vi "Window-Export time series snippet.vi"(10 "New folder path":path, 11 "Existing AVI path":path) -> ()   [LabVIEW 2017]
uses:
  <vilib>/Utility/miscctls.llb/LVPointTypeDef.ctl
panel:
  out "Ended":bool
  out "Manually closed":bool
  out "Exporting snippet...":u8(slide) scale=0.0..100.0
  out "# of Frames in exported portion":i32 format="Number of frames: %.0f"
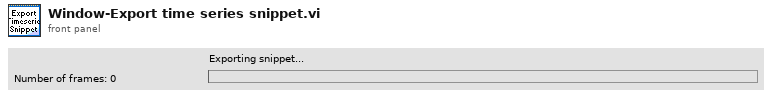
[diagram p1: front panel]
types:
  T1 = typedef "Image Type" = u32
  T2 = typedef "LVPointTypeDef.ctl" = cluster{"Horizontal":i16, "Vertical":i16}
  T3 = typedef "AVI modes refs cluster.ctl" = cluster{"AVI1 ref":T4, "AVI2 refs":T5[], "AVI # frames":u32[]}
  T4 = typedef "AviRefnum.ctl" = refnum<k1>
  T5 = typedef "IMAQ AVI2 Refnum.ctl" = refnum<k20>
  T6 = typedef "Fixed strings.ctl" = cluster{"ROI file name":string, "Normalised ROI file name":string, "Zplane Pockels values file name":string, "Functional data folder name":string, "Experiment Header file name":string, "Z-stack images folder name":string, "Groups setup rel. path":string, "Groups text file rel. path":string, "TDMS files folder name (F.img)":string, "TDMS files folder name (V.acq)":string, "TDMS files folder name (Pl.acq)":string, "Cycle rel times sequence file":string, "Dynamically called VIs folder name":string, "Time Series folder base name":string}
  T7 = typedef "IMAQ Image.ctl" = refnum<image>
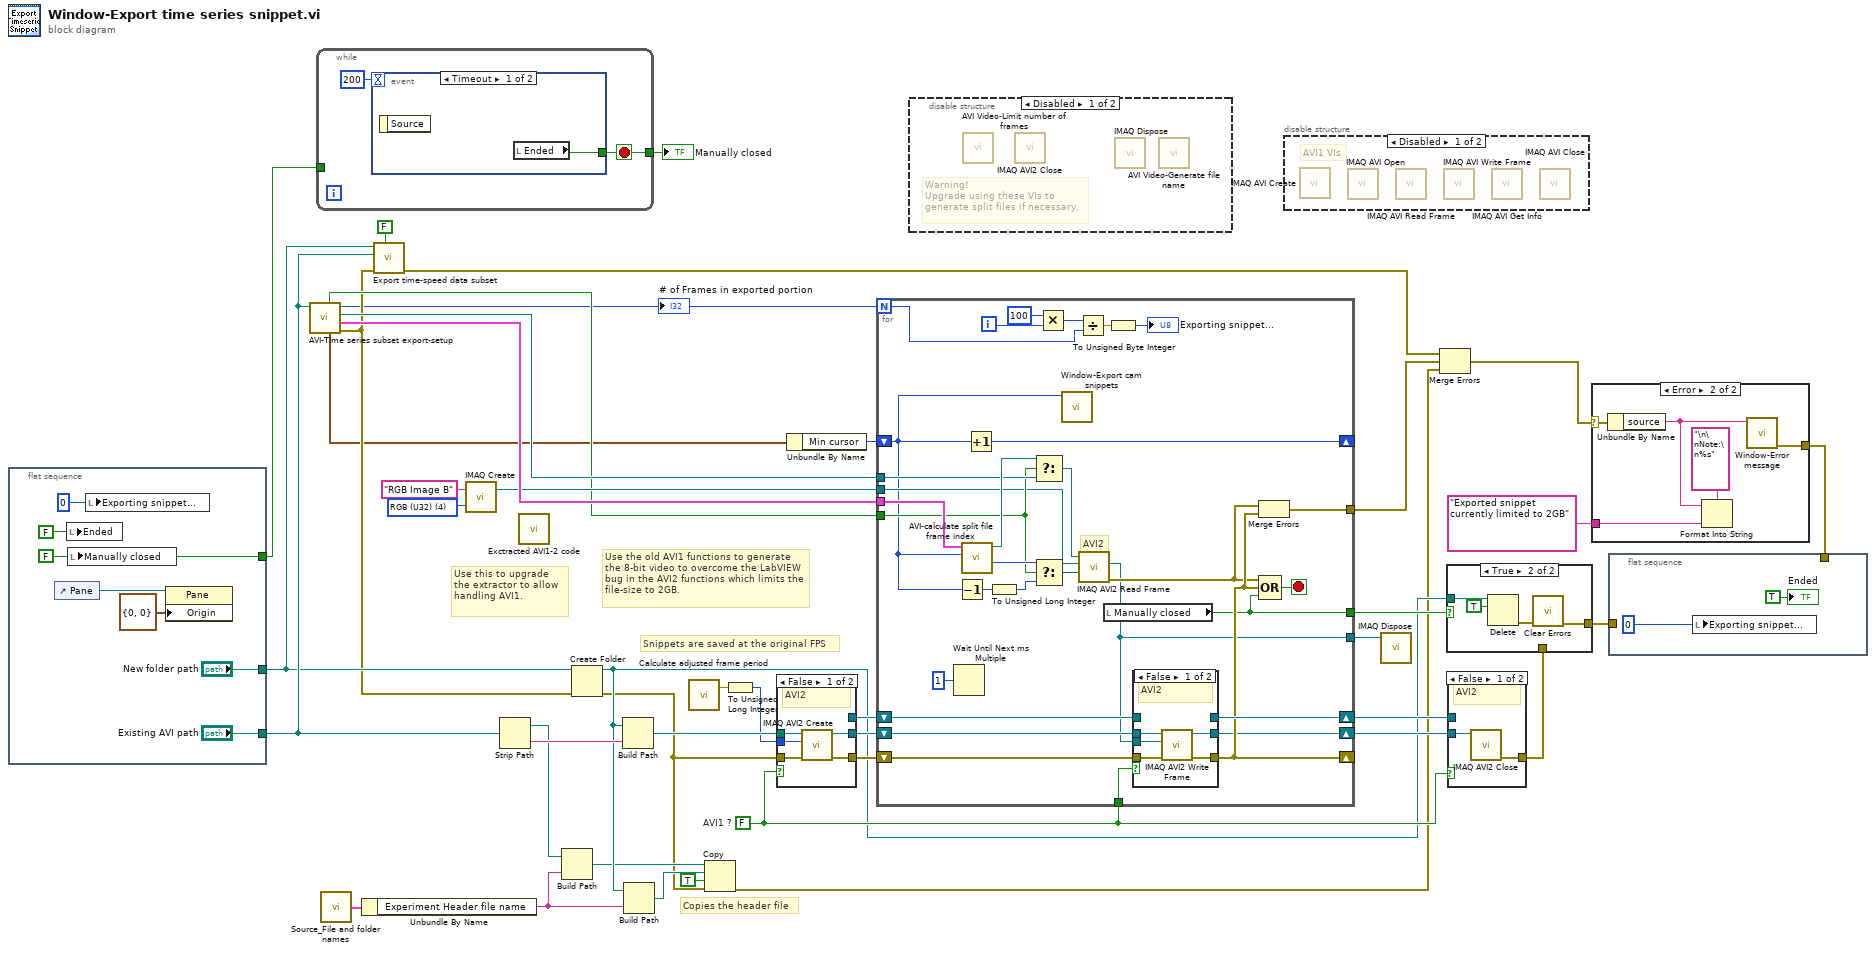
[diagram p0: block diagram]
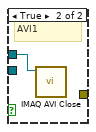
[diagram p4: hidden frame]
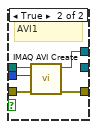
[diagram p5: hidden frame]
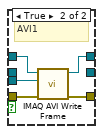
[diagram p6: hidden frame]
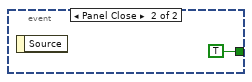
[diagram p8: hidden frame]
diagram:
  w30 = FALSE  # AVI1 ?
  w41 = T1 4 items=["Grayscale (U8)", "Grayscale (I16)", "Grayscale (SGL)", "Complex (CSG)", "RGB (U32)", "HSL (U32)", "RGB (U64)", "Grayscale (U16)"] ("Image Type")
  # "Snippets are saved at the original FPS"
  # "Use this to upgrade the extractor to allow handling AVI1."
  # "Copies the header file"
  # "Use the old AVI1 functions to generate the 8-bit video to overcome the LabVIEW bug in the AVI2 functions which limits the file-size to 2GB."
  n1 = flat-sequence {
    tunnel: ["Existing AVI path"] -> w11
    tunnel: ["New folder path"] -> w10
    tunnel: [w48] -> w42
    frame #0 {
      w48 = FALSE
      n2 = control-ref of="Pane"() -> (w44:refnum<vi>)
      n3 = local write "Ended"(FALSE) -> ()
      n4 = local write "Manually closed"(w48) -> ()
      n5 = local write "Exporting snippet..."(u8 0 ("Progress...")) -> ()
      n6 = property class="Pane"(reference=w44, "Origin"=T2 {"Horizontal"=0, "Vertical"=0}) -> ()  [unwired: 1 in, 2 out]
    }
  }
  n7 = call "AVI-Time series subset export-setup.vi"("AVI path & name"=w11) -> ("error out"=w9:errorcluster, "AVI modes refs"=w39:T3, "AVI Refnum (duplicate)"=w37:T5, "# of Frames in exported portion"=w7:i32, "Extraction cursors"=w6:cluster{"Min cursor":i32, "Max cursor":i32}, "Export all split AVI files as one"=w16:bool)  [unwired: 5 in]
  "# of Frames in exported portion" <- w7
  n8 = while {
    tunnel: [w51] -> w43
    tunnel: w42 -> [_]
    stop <- w51 stop-if-true
    n9 = event shown="[0] Timeout" {
      selector: _ -> [_ _]
      dyn-events: _ -> [_ _]
      timeout: 200 -> [_ _]
      tunnel: [w53 TRUE] -> w51
      event Timeout {
        n10 = event-data() -> ()  [unwired: 1 in, 1 out]
        n11 = local read "Ended"() -> (w53:bool)
      }
      event Panel Close {
        n12 = event-data() -> ()  [unwired: 1 in, 1 out]
      }
    }
  }
  "Manually closed" <- w43
  n13 = call "Source_File and folder names.vi"() -> ("Fixed strings"=w5:T6)  [unwired: 1 in]
  n14 = Unbundle By Name(w5) -> ("Experiment Header file name"=w4:string)
  n15 = call "Export time-speed data subset.vi"("Funct data structure"=FALSE, "error in (no error)"=w9, "Existing AVI path"=w11, "New folder path"=w10) -> ("error out"=w8:errorcluster)  [unwired: 5 in, 2 out]
  n16 = call "IMAQ Create"("Image Name"="RGB Image B", "Image Type"=w41) -> ("New Image"=w38:T7)  [unwired: 2 in, 2 out]
  n17 = Strip Path(path=w11) -> (stripped path=w23:path, name=w25:string)
  n18 = call "Exctracted AVI1-2 code.vi"() -> ()  [unwired: 12 in]
  n19 = Build Path(base path=w23, name or relative path=w4) -> (appended path=w22:path)
  n20 = Create Folder(path (use dialog)=w10, error in=w9) -> (created path=w24:path, error out=w15:errorcluster)  [unwired: 1 in, 1 out]
  n21 = Build Path(base path=w24, name or relative path=w25) -> (appended path=w33:path)
  n22 = Build Path(base path=w24, name or relative path=w4) -> (appended path=w21:path)
  n23 = call "Calculate adjusted frame period.vi"() -> ("Original frame rate (fps)"=w3:dbl)  [unwired: 9 in, 2 out]
  n24 = Copy(8:w15, 9:TRUE ("overwrite (F)"), 10:w21, 11:w22) -> (0:w14:errorcluster)  [unwired: 1 in, 2 out]
  n25 = To Unsigned Long Integer(number=w3) -> (unsigned 32bit integer=w2:u32)
  n26 = case shown="False" w30 {
    tunnel: [_ w64] -> w35
    tunnel: [w59 w63] -> w34
    tunnel: w33 -> [w58 w62]
    tunnel: w2 -> [w57 w61]
    tunnel: [w56 _] -> w32
    tunnel: w15 -> [w55 w60]
    frame False {
      # "AVI2"
      n27 = call "IMAQ AVI2 Create"("error in (no error)"=w55, "Frames Per Second"=w57, "AVI Path"=w58) -> ("error out"=w59:errorcluster, "AVI Refnum"=w56:T5)  [unwired: 7 in]
    }
    frame True {
      # "AVI1"
      n28 = call "IMAQ AVI Create"("error in (no error)"=w60, "Frames Per Second"=w61, "AVI Path"=w62) -> ("error out"=w63:errorcluster, "Avi Refnum"=w64:T4)  [unwired: 7 in]
    }
  }
  n29 = Unbundle By Name(w6) -> ("Min cursor"=w29:i32)
  n30 = for {
    N: w7 -> [w75]
    tunnel: w37 -> [w88]
    tunnel: w38 -> [w73]
    shift-right: [w95] -> w36
    shift-left: w35 -> [w94]
    shift-right: [w92] -> _
    shift-left: w34 -> [w93]
    tunnel: [w91] -> w12
    tunnel: w39 -> [w90]
    tunnel: w16 -> [w86]
    shift-right: [w79] -> w31
    shift-left: w32 -> [w80]
    tunnel: w30 -> [w78]
    shift-right: [w74] -> _
    shift-left: w29 -> [w65]
    tunnel: [w69] -> w28
    tunnel: [w66] -> w27
    i -> [w67]
    stop <- w85 stop-if-true
    # "AVI2"
    n31 = Wait Until Next ms Multiple(millisecond multiple=u32 1) -> ()  [unwired: 1 out]
    n32 = Decrement(x=w65) -> (x-1=w77:i32)
    n33 = call "AVI-calculate split file frame index.vi"("Frame number (unity-based) in"=w65, "AVI modes refs"=w90) -> ("Index of frame in split file"=w87:u32, "AVI2 split file ref"=w89:T5)  [unwired: 6 in, 2 out]
    n34 = Increment(x=w65) -> (x+1=w74:i32)
    n35 = To Unsigned Long Integer(number=w77) -> (unsigned 32bit integer=w76:u32)
    n36 = Select(t=w89, s=w86, f=w88) -> (s? t:f=w72:T5)
    n37 = Select(t=w87, s=w86, f=w76) -> (s? t:f=w71:u32)
    n38 = Multiply(x=100, y=w67) -> (x*y=w83:i32)
    n39 = call "Window-Export cam snippets.vi"("Min cursor"=w65) -> ()  [unwired: 11 in]
    n40 = Divide(x=w83, y=w75) -> (x/y=w82:dbl)
    n41 = call "IMAQ AVI2 Read Frame"("Frame Number"=w71, "Image"=w73, "AVI Refnum"=w72) -> ("error out"=w70:errorcluster, "Image Out"=w69:T7)  [unwired: 6 in, 1 out]
    n42 = local read "Manually closed"() -> (w66:bool)
    n43 = To Unsigned Byte Integer(number=w82) -> (unsigned 8bit integer=→"Exporting snippet...":u8)
    n44 = case shown="False" w78 {
      tunnel: [_ w105] -> w95
      tunnel: w94 -> [_ w104]
      tunnel: w93 -> [w100 w103]
      tunnel: [w99 w102] -> w92
      tunnel: w69 -> [w96 w101]
      tunnel: w80 -> [w98 _]
      tunnel: [w97 _] -> w79
      frame False {
        # "AVI2"
        n45 = call "IMAQ AVI2 Write Frame"("error in (no error)"=w100, "Image"=w96, "AVI Refnum"=w98) -> ("error out"=w99:errorcluster, "AVI Refnum (duplicate)"=w97:T5)  [unwired: 6 in, 1 out]
      }
      frame True {
        # "AVI1"
        n46 = call "IMAQ AVI Write Frame"("error in (no error)"=w103, "Image"=w101, "Avi Refnum"=w104) -> ("error out"=w102:errorcluster, "Avi Refnum (duplicate)"=w105:T4)  [unwired: 7 in]
      }
    }
    n47 = Merge Errors(w70, w92) -> (w91:errorcluster)
    n48 = Compound Arithmetic op=OR(w70, w92, w66) -> (w85:bool)
  }
  n49 = disable-structure shown="Disabled" {
    frame Disabled {
      # "Warning!\nUpgrade using these VIs to \ngenerate split files if necessary."
      n50 = call "AVI Video-Limit number of frames.vi"() -> ()  [unwired: 1 in, 1 out]
      n51 = call "IMAQ AVI2 Close"() -> ()  [unwired: 11 in, 1 out]
      n52 = call "IMAQ Dispose"() -> ()  [unwired: 6 in, 1 out]
      n53 = call "AVI Video-Generate file name.vi"() -> ()  [unwired: 10 in, 2 out]
    }
    frame Enabled {
    }
  }
  n54 = disable-structure shown="Disabled" {
    frame Disabled {
      # "AVI1 VIs"
      n55 = call "IMAQ AVI Create"() -> ()  [unwired: 10 in, 2 out]
      n56 = call "IMAQ AVI Open"() -> ()  [unwired: 10 in, 2 out]
      n57 = call "IMAQ AVI Read Frame"() -> ()  [unwired: 8 in, 4 out]
      n58 = call "IMAQ AVI Write Frame"() -> ()  [unwired: 10 in, 2 out]
      n59 = call "IMAQ AVI Get Info"() -> ()  [unwired: 7 in, 5 out]
      n60 = call "IMAQ AVI Close"() -> ()  [unwired: 11 in, 1 out]
    }
    frame Enabled {
    }
  }
  n61 = call "IMAQ Dispose"("Image"=w28) -> ()  [unwired: 5 in, 1 out]
  n62 = Merge Errors(w8, w12, w14) -> (w13:errorcluster)
  n63 = case shown="False" w30 {
    tunnel: w36 -> [_ w108]
    tunnel: w31 -> [w107 _]
    tunnel: [w106 _] -> w26
    frame False {
      # "AVI2"
      n64 = call "IMAQ AVI2 Close"("AVI Refnum"=w107) -> ("error out"=w106:errorcluster)  [unwired: 10 in]
    }
    frame True {
      # "AVI1"
      n65 = call "IMAQ AVI Close"("Avi Refnum"=w108) -> ()  [unwired: 10 in, 1 out]
    }
  }
  n66 = case shown="True" w27 {
    tunnel: w24 -> [_ w112]
    tunnel: w26 -> [_ _]
    tunnel: [_ w109] -> w19
    frame False {
    }
    frame True {
      n67 = Delete(path (use dialog)=w112, entire hierarchy (F)=TRUE) -> (error out=w111:errorcluster)  [unwired: 3 in, 2 out]
      n68 = call <vilib>:"Clear Errors.vi"("error in (no error)"=w111) -> ("error out"=w109:errorcluster)  [unwired: 5 in, 1 out]
    }
  }
  n69 = case shown="Error" w13 {
    selector: w13 -> [_ w117]
    tunnel: [_ w116] -> w17
    tunnel: "Exported snippet currently limited to 2GB" ("message") -> [_ w113]
    frame No Error {
    }
    frame Error {
      n70 = Unbundle By Name(w117) -> ("source"=w114:string)
      n71 = Format Into String(format string="\n\nNote:\n%s", initial string=w114, w113) -> ()  [unwired: 1 in, 2 out]
      n72 = call "Window-Error message.vi"("Message"=w114) -> ("Error Out (no error)"=w116:errorcluster)  [unwired: 10 in]
    }
  }
  n73 = flat-sequence {
    tunnel: w19 -> [_]
    tunnel: w17 -> [_]
    frame #0 {
      n74 = local write "Exporting snippet..."(u8 0 ("Progress...")) -> ()
      "Ended" <- TRUE ("Ended")
    }
  }
